vi "Update Pot Button Text.vi"(8 "error in":errorcluster, 11 "Button Reference":refnum<vi>) -> (0 "error out":errorcluster, 2 "Value":bool)   [LabVIEW 2017]
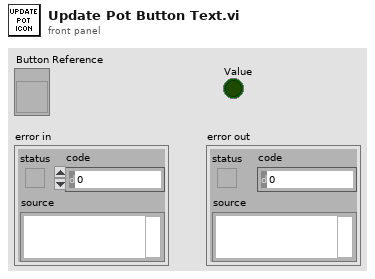
[diagram p1: front panel]
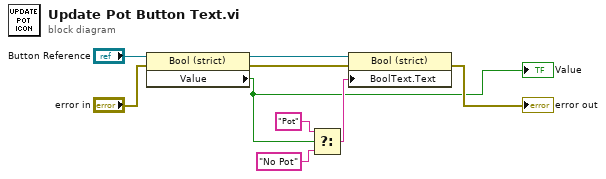
[diagram p0: block diagram]
diagram:
  n1 = property class="Bool (strict)"(reference="Button Reference", error in="error in") -> (reference out=w4:refnum<vi>, error out=w3:errorcluster, "Value"=w1:bool)
  "Value" <- w1
  n2 = Select(t="Pot", s=w1, f="No Pot") -> (s? t:f=w7:string)
  n3 = property class="Bool (strict)"(reference=w4, error in=w3, "BoolText.Text"=w7) -> (error out=→"error out":errorcluster)  [unwired: 1 out]
